vi "ROSPublisher.vi"(2 "Response":T1, 3 "ROS":T2={"topic port"=1236, "Node"="/labview", "topic"="/robot/head/command_head_nod", "type"="std_msgs/Bool", "node port"=7000, "error "={"status"=FALSE, "code"=0, "source"=""}, "Direction"=enum."Publisher", "Update (ms)"=1, "FIFO size"=1}) -> ()   [LabVIEW 2015]
uses:
  SubVIs/_ROSControl.ctl
  SubVIs/_ROSDirection.ctl
  Console/Servers/ServerSubs/ROSLog.ctl
  _ROSDefinition.vi
panel:
  out "ports":i32[](array[numeric])
  out "Queue log":string
  out "Watchdog":i32
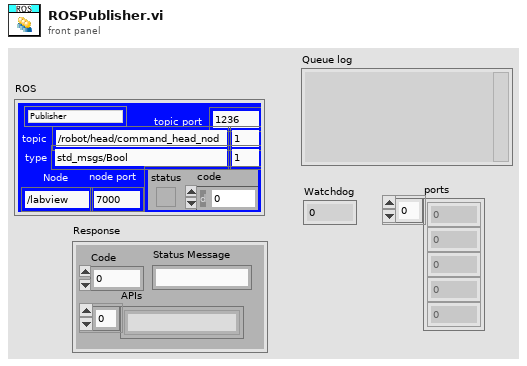
[diagram p1: front panel]
types:
  T1 = cluster{"Code":i32, "Status Message":string, "APIs":string[]}
  T2 = typedef "_ROSControl.ctl" = cluster{"topic port":u16, "Node":string, "topic":string, "type":string, "node port":u16, "error ":errorcluster, "Direction":T3, "Update (ms)":u16, "FIFO size":u16}
  T3 = typedef "_ROSDirection.ctl" = enum16{"Node", "Publisher", "Subscriber", "ServiceClient", "ServiceProvider"}
  T4 = enum16{"Reset Log", "Add Client", "Remove Client", "Add Task"}
  T5 = typedef "ROSLog.ctl" = cluster{"Sent":string, "Reply":string, "MethodName":string, "success":bool, "Dir1":string, "Dir2":string, "Time Stamp":string, "error":errorcluster, "Preamble":string, "Midamble":string, "Postamble":string}
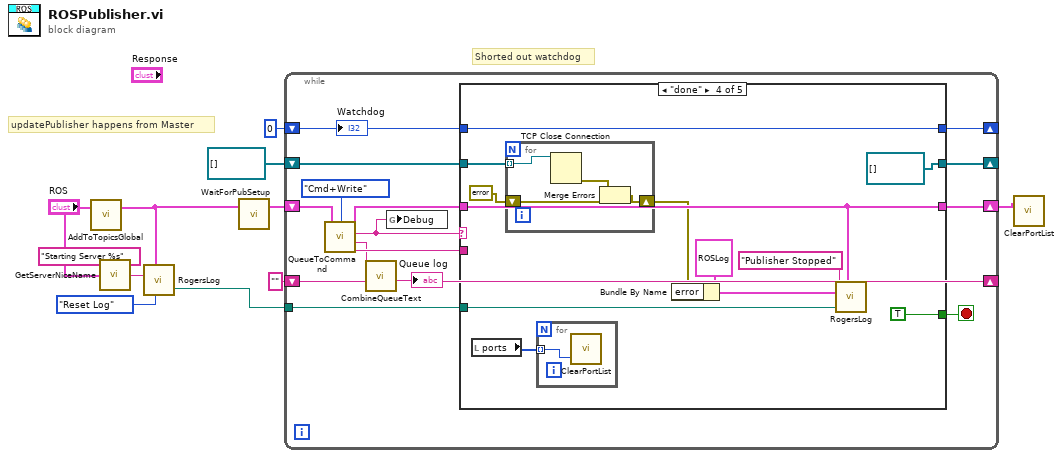
[diagram p0: block diagram]
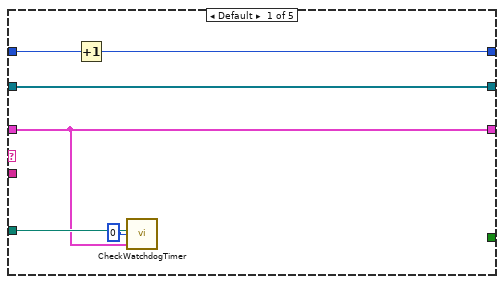
[diagram p2: hidden frame]
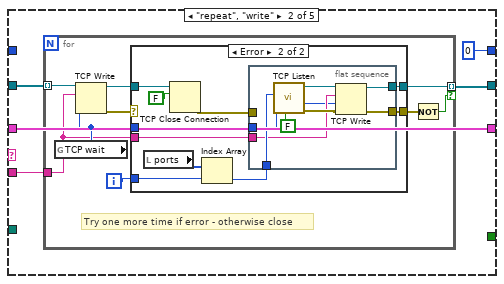
[diagram p3: hidden frame]
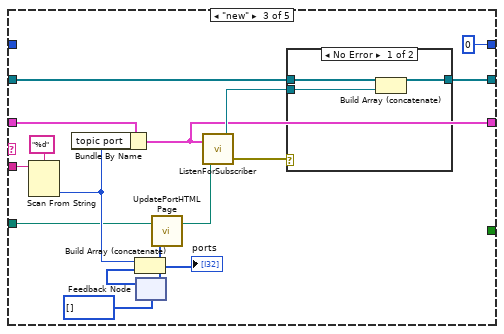
[diagram p5: hidden frame]
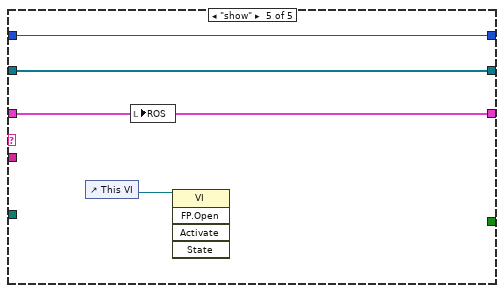
[diagram p7: hidden frame]
diagram:
  # "Shorted out watchdog"
  # "updatePublisher happens from Master"
  n1 = call "AddToTopicsGlobal.vi"("ROS in"="ROS") -> ("ROS out"=w1:T2)  [unwired: 2 in]
  n2 = call "GetServerNiceName.vi"("ROS"="ROS", "Text to add"="Starting Server %s") -> ("String"=w10:string)
  n3 = call "RogersLog.vi"("Text to add"=w10, "ROS"=w1, "Task"=T4."Reset Log") -> ("LogPath out"=w7:path)  [unwired: 2 in, 1 out]
  n4 = call "WaitForPubSetup.vi"("ROS in"=w1) -> ("ROS out"=w5:T2)  [unwired: 2 in]
  n5 = while {
    tunnel: w7 -> [w23]
    shift-right: [w21] -> _
    shift-left: 0 ("timeout ms (wait forever: -1)") -> [w22]
    shift-right: [w20] -> _
    shift-left: refnum<k5>[] [] -> [w26]
    shift-right: [w17] -> _
    shift-left: "" ("New List") -> [w19]
    shift-right: [w14] -> w2
    shift-left: w5 -> [w16]
    stop <- w24 stop-if-true
    n6 = call "QueueToCommand.vi"("ROS"=w16, "Check"=enum16{"Cmd+Write", "FIFO", "CMD", "CMD /wait"}."Cmd+Write") -> ("ROS out"=w15:T2, "Command"=w12:string, "Queue log"=w18:string, "data"=w25:string)  [unwired: 1 in]
    n7 = call "CombineQueueText.vi"("Old List"=w19, "Queue In"=w18) -> ("New List"=w17:string)  [unwired: 1 in]
    "Queue log" <- w17
    n8 = global write "_ROSDefinition.vi" "Debug"(w12) -> ()
    n9 = case shown="\"done\"" w12 {
      tunnel: w26 -> [w31 w36 w78 w92 w104]
      tunnel: w25 -> [_ w33 w80 _ _]
      tunnel: [_ _ _ TRUE _] -> w24
      tunnel: w23 -> [w29 _ w69 w96 _]
      tunnel: w22 -> [w32 _ _ w94 w105]
      tunnel: [w30 0 ("timeout ms (wait forever: -1)") 0 ("timeout ms (wait forever: -1)") w94 w105] -> w21
      tunnel: w15 -> [w27 w34 w71 w90 w103]
      tunnel: [w31 w35 w76 refnum<k5>[] [] w104] -> w20
      tunnel: [w27 w34 w67 w90 w103] -> w14
      frame Default {
        n10 = Increment(x=w32) -> (x+1=w30:i32)
        n11 = call "CheckWatchdogTimer.vi"("ROS"=w27, "itteration"=0, "LogPath in"=w29) -> ()  [unwired: 3 in]
      }
      frame "repeat", "write" {
        n12 = for {
          tunnel: w36 -> [w46] mode=indexing
          tunnel: w33 -> [w40]
          tunnel: [w43] -> w35 mode=indexing if=w38
          i -> [w42]
          # "Try one more time if error - otherwise close"
          n13 = global read "_ROSDefinition.vi" "TCP wait"() -> (w41:i32)
          n14 = TCP Write(connection ID=w46, data in=w40, 9:w41) -> (connection ID out=w44:refnum<k5>, error out=w45:errorcluster)  [unwired: 1 in, 1 out]
          n15 = case shown="Error" w45 {
            selector: w45 -> [w47 _]
            tunnel: w44 -> [w48 w58]
            tunnel: [w48 w56] -> w43
            tunnel: w42 -> [_ w54]
            tunnel: w41 -> [_ w51]
            tunnel: w40 -> [_ w50]
            tunnel: [w47 w49] -> w39
            frame No Error {
            }
            frame Error {
              n16 = local read "ports"() -> (w55:i32[])
              n17 = TCP Close Connection(connection ID=w58, abort (F)=FALSE) -> (error out=w52:errorcluster)  [unwired: 1 in, 1 out]
              n18 = Index Array(array=w55, index=w54) -> (element=w53:i32)
              n19 = flat-sequence {
                tunnel: [w62] -> w56
                tunnel: w53 -> [w66]
                tunnel: w51 -> [w59]
                tunnel: w52 -> [_]
                tunnel: [w64] -> w49
                tunnel: w50 -> [w61]
                frame #0 {
                  n20 = call "TCP Listen.vi"("resolve remote address (T)"=FALSE, "timeout ms (wait forever: -1)"=w59, "port"=w66) -> ("error out"=w65:errorcluster, "connection ID"=w63:refnum<k5>)  [unwired: 4 in, 3 out]
                  n21 = TCP Write(connection ID=w63, data in=w61, error in (no error)=w65, 9:w59) -> (connection ID out=w62:refnum<k5>, error out=w64:errorcluster)  [unwired: 1 out]
                }
              }
            }
          }
          n22 = Not(x=w39) -> (.not. x?=w38:bool)
        }
      }
      frame "new" {
        n23 = Scan From String(format string="%d", input string=w80) -> (output 1=w74:i32)  [unwired: 3 in, 3 out]
        n24 = Bundle By Name(cluster=w71, "topic port"=w74) -> (w67:T2)
        n25 = feedback #1(i32[] []) -> (w73:i32[])
        n26 = Build Array (concatenate)(w74, w73) -> (w68:i32[])
        "ports" <- w68
        n27 = feedback-in #1(w68) -> ()
        n28 = call "UpdatePortHTMLPage.vi"("Array"=w68, "LogPath in"=w69) -> ("LogPath out"=w70:path)  [unwired: 1 in]
        n29 = call "ListenForSubscriber.vi"("LogPath in"=w70, "ROS"=w67) -> ("heard?"=w75:errorcluster, "server"=w77:refnum<k5>)
        n30 = case shown="No Error" w75 {
          tunnel: w78 -> [w84 w85]
          tunnel: w77 -> [w83 _]
          tunnel: [w82 w85] -> w76
          frame No Error {
            n31 = Build Array (concatenate)(w84, w83) -> (w82:refnum<k5>[])
          }
          frame Error {
          }
        }
      }
      frame "done" {
        n32 = local read "ports"() -> (w93:i32[])
        n33 = for {
          tunnel: w92 -> [w101] mode=indexing
          shift-right: [w99] -> w86
          shift-left: errorcluster {"status"=FALSE, "code"=0, "source"=""} ("error IO") -> [w98]
          n34 = TCP Close Connection(connection ID=w101) -> (error out=w100:errorcluster)  [unwired: 2 in, 1 out]
          n35 = Merge Errors(w100, w98) -> (w99:errorcluster)
        }
        n36 = for {
          tunnel: w93 -> [w102] mode=indexing
          n37 = call "ClearPortList.vi"("topic port"=w102) -> ()  [unwired: 2 in]
        }
        n38 = Bundle By Name(cluster=T5 {"Sent"="", "Reply"="", "MethodName"="", "success"=TRUE, "Dir1"="", "Dir2"="", "Time Stamp"="", "error"={"status"=FALSE, "code"=0, "source"=""}, "Preamble"="", "Midamble"="", "Postamble"=""} ("Log"), "error"=w86) -> (w88:T5)
        n39 = call "RogersLog.vi"("Text to add"="Publisher Stopped", "ROS"=w90, "Log"=w88, "LogPath in"=w96) -> ()  [unwired: 1 in, 2 out]
      }
      frame "show" {
        n40 = control-ref of="This VI"() -> (w106:refnum<vi>)
        n41 = local write "ROS"(w103) -> ()
        n42 = invoke class="VI" method="FP.Open"(reference=w106) -> ()  [unwired: 4 in, 5 out]
      }
    }
    "Watchdog" <- w22
  }
  n43 = call "ClearPortList.vi"("ROS"=w2) -> ()  [unwired: 2 in]
